vi "TestChar2.vi"() -> ()   [LabVIEW 2014]
panel:
  out "ChartOut":picture
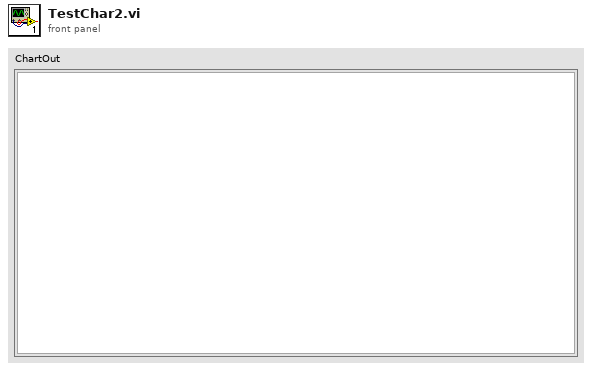
[diagram p1: front panel]
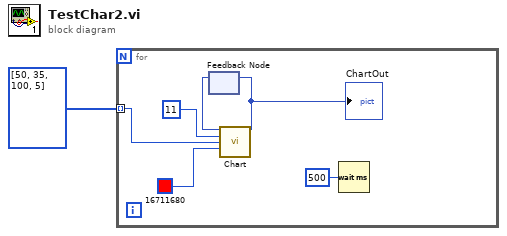
[diagram p0: block diagram]
diagram:
  n1 = for {
    tunnel: i32[] [50, 35, 100, 5] -> [w5] mode=indexing
    n2 = feedback #1() -> (w6:picture)  [unwired: 1 in]
    n3 = call "Chart.vi"("PictureIn"=w6, "x"=i16 11, "y"=w5, "colorRectangle"=u32 16711680) -> ("ChartOut"=w7:picture)  [unwired: 10 in, 1 out]
    "ChartOut" <- w7
    n4 = feedback-in #1(w7) -> ()
    n5 = Wait (ms)(milliseconds to wait=u32 500) -> ()  [unwired: 1 out]
  }
